vi "SLL DE Virtual Graph Channel Parameters.vi"(8 "error in (no error)":errorcluster, 11 "Virtual Channel Name":string="None") -> (0 "error out":errorcluster, 1 "Maximum Value":dbl, 2 "Minimum Value":dbl, 3 "Graph Name Label":string, 4 "Increment":dbl, 5 "Channel Type":T1)   [LabVIEW 2013]
doc: "Copyright © 2005, Soliton Technologies.\nAll rights reserved."
uses:
  Sub VIs/DAQ Engine/Controls/SLL DE Unit Info LV2Global Options.ctl
  Sub VIs/DAQ Engine/Controls/SLL DE List of AI Channel Type.ctl
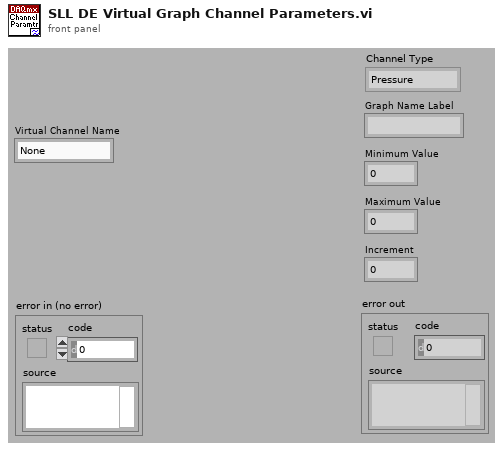
[diagram p1: front panel]
types:
  T1 = typedef "SLL DE List of AI Channel Type.ctl" = enum16{"Pressure", "Flow", "Temperature", "Time Scale", "Voltage", "Current", "Frequency", "Sound", "Speed", "Torque", "Distance", "Channel Type 1", "Channel Type 2", "Channel Type 3"}
  T2 = typedef "SLL DE Unit Info LV2Global Options.ctl" = enum16{"Update Channel Type", "Update Unit Info", "Get Unit Info", "Read"}
  T3 = cluster{"Channel Type":T1, "Unit Text":string, "Maximum":dbl, "Minmum":dbl, "Increments":dbl}
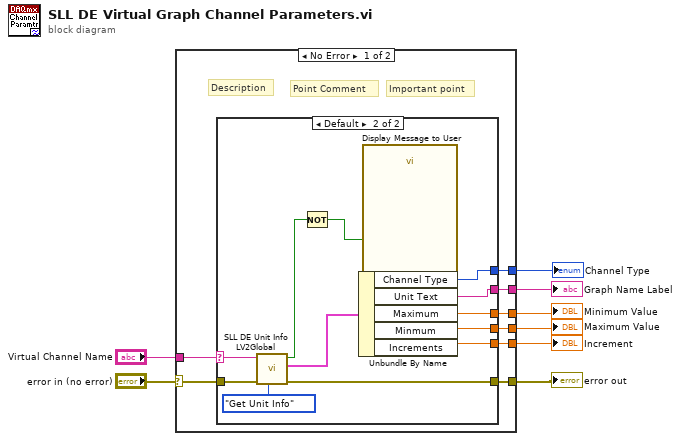
[diagram p0: block diagram]
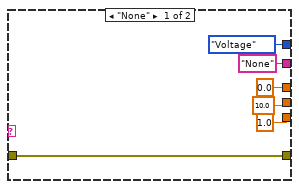
[diagram p2: hidden frame]
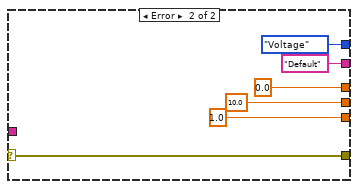
[diagram p3: hidden frame]
diagram:
  n1 = case shown="No Error" "error in (no error)" {
    selector: "error in (no error)" -> [w16 w40]
    tunnel: [w15 w40] -> w6
    tunnel: "Virtual Channel Name" -> [w9 _]
    tunnel: [w14 1.0 ("Increments")] -> w5
    tunnel: [w13 10.0 ("Minmum")] -> w4
    tunnel: [w12 0.0 ("Maximum")] -> w3
    tunnel: [w11 "Default" ("Unit Text")] -> w2
    tunnel: [w10 SLL_DE_List_of_AI_Channel_Type."Voltage" ("Channel Type")] -> w1
    frame No Error {
      # "Point Comment"
      # "Important point"
      # "Description"
      n2 = case shown="Default" w9 {
        selector: w9 -> [_ w23]
        tunnel: w16 -> [w17 w32]
        tunnel: [w17 w31] -> w15
        tunnel: [1.0 ("Increments") w30] -> w14
        tunnel: [10.0 ("Minmum") w29] -> w13
        tunnel: [0.0 ("Maximum") w28] -> w12
        tunnel: ["None" ("Unit Text") w27] -> w11
        tunnel: [SLL_DE_List_of_AI_Channel_Type."Voltage" ("Channel Type") w24] -> w10
        frame "None" {
        }
        frame Default {
          n3 = call "SLL DE Unit Info LV2Global.vi"("Option"=SLL_DE_Unit_Info_LV2Global_Options."Get Unit Info", "Error in (no error)"=w32, "Channel Name"=w23) -> ("Error out"=w31:errorcluster, "Unit Info"=w33:T3, "Valid?"=w26:bool)  [unwired: 6 in]
          n4 = Not(x=w26) -> (.not. x?=w25:bool)
          n5 = Unbundle By Name(w33) -> ("Channel Type"=w24:T1, "Unit Text"=w27:string, "Maximum"=w28:dbl, "Minmum"=w29:dbl, "Increments"=w30:dbl)
          n6 = call "Display Message to User"("Enable"=w25) -> ()  [unwired: 9 in, 2 out]
        }
      }
    }
    frame Error {
    }
  }
  "error out" <- w6
  "Graph Name Label" <- w2
  "Minimum Value" <- w3
  "Maximum Value" <- w4
  "Increment" <- w5
  "Channel Type" <- w1
